vi "Assert Service Location.vi"(8 "expected unique id":u64, 9 "actual unique id":u64, 10 "expected service location port":string="0", 11 "actual service location":T1) -> (2 "result":string, 3 "pass":bool)   [LabVIEW 2020, in "MeasurementServerTests.lvlib" / "gRPC Utilities Tests.lvlib"]
uses:
  gRPC Utilities Tests.lvlib
  Runtime/MeasurementLink Discovery Client/RPC Messages/ni_measurementlink_discovery_v1_ServiceLocation.ctl
  Runtime/MeasurementLink Discovery Client/MeasurementLink Discovery Client.lvlib
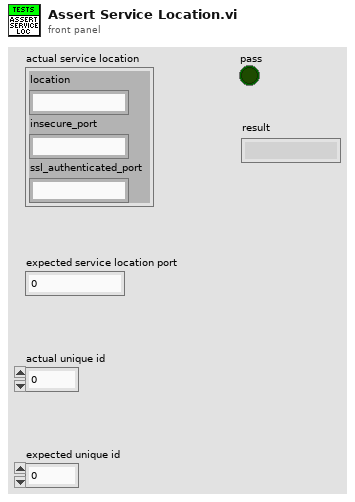
[diagram p1: front panel]
types:
  T1 = typedef "MeasurementLink Discovery Client.lvlib/ni_measurementlink_discovery_v1_ServiceLocation.ctl" = cluster{"location":string, "insecure_port":string, "ssl_authenticated_port":string}
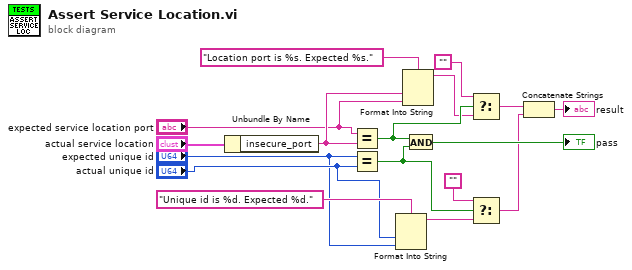
[diagram p0: block diagram]
diagram:
  n1 = Unbundle By Name("actual service location") -> ("insecure_port"=w14:string)
  n2 = Equal?(x="expected service location port", y=w14) -> (x = y?=w12:bool)
  n3 = Equal?(x="expected unique id", y="actual unique id") -> (x = y?=w6:bool)
  n4 = Format Into String(format string="Unique id is %d. Expected %d.", "actual unique id", "expected unique id") -> (resulting string=w5:string)  [unwired: 2 in, 1 out]
  n5 = Format Into String(format string="Location port is %s. Expected %s.", w14, "expected service location port") -> (resulting string=w11:string)  [unwired: 2 in, 1 out]
  n6 = And(x=w12, y=w6) -> (x .and. y?=→"pass":bool)
  n7 = Select(t="", s=w12, f=w11) -> (s? t:f=w10:string)
  n8 = Select(t="", s=w6, f=w5) -> (s? t:f=w2:string)
  n9 = Concatenate Strings(w10, w2) -> (→"result":string)
